vi "FTW-JSON-SetFlags-Encoding.vi"(0 "JSON Object":refnum<data-value>, 5 "Indent Spaces":i32=4, 7 "Escape Unicode":bool=TRUE, 9 "Sort Keys":bool, 11 "error in":errorcluster, 12 "Floating Point Significant Digits":i32=16) -> (4 "JSON Object out":refnum<data-value>, 15 "error out":errorcluster)   [LabVIEW 2014]
uses:
  core/FTW-JSON-Core-Structure.ctl
panel:
  # "Inputs"
  # "Outputs"
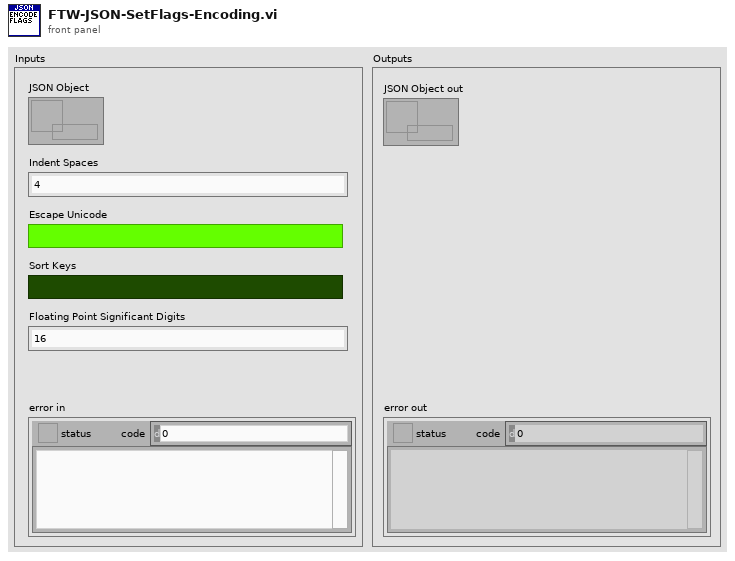
[diagram p1: front panel]
types:
  T1 = typedef "FTW-JSON-Core-Structure.ctl" = cluster{"JSON Object":i64, "Encoding Flags":i64, "Decoding Flags":i64}
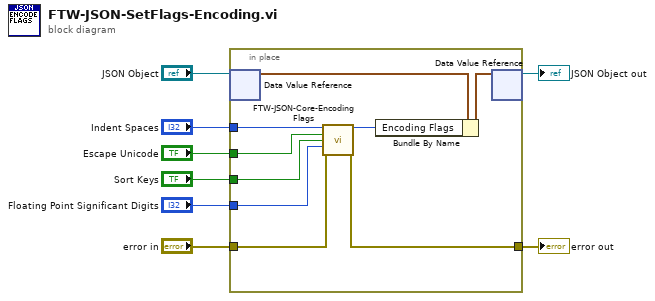
[diagram p0: block diagram]
diagram:
  n1 = in-place {
    in-place-border: "Indent Spaces" -> [w17]
    in-place-border: "Escape Unicode" -> [w16]
    in-place-border: "Sort Keys" -> [w15]
    in-place-border: "Floating Point Significant Digits" -> [w14]
    in-place-border: "error in" -> [w12]
    in-place-border: [w11] -> w3
    n2 = in-place-dvr #1("JSON Object") -> (w10:T1)  [unwired: 1 out]
    n3 = call "FTW-JSON-Core-EncodingFlags.vi"("Indent Spaces"=w17, "Escape Unicode"=w16, "Sort Keys"=w15, "Floating Point Significant Digits"=w14, "error in"=w12) -> ("Encoding Flags"=w13:i64, "error out"=w11:errorcluster)  [unwired: 9 in]
    n4 = Bundle By Name(cluster=w10, "Encoding Flags"=w13) -> (w9:T1)
    n5 = in-place-dvr #1(w9) -> (→"JSON Object out":refnum<data-value>)  [unwired: 1 out]
  }
  "error out" <- w3
